vi "CAMERA ROI.vi"(8 "error in (no error)":errorcluster, 11 "Enum":T1=enum."INIT") -> (0 "error out":errorcluster)   [LabVIEW 2025]
uses:
  POST ANALYSIS ENUM.ctl
panel:
  in  "stop":bool
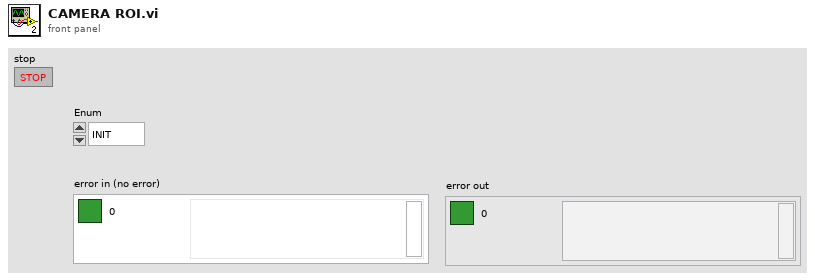
[diagram p1: front panel]
types:
  T1 = typedef "POST ANALYSIS ENUM.ctl" = enum16{"OPEN EXE", "INIT", "OPEN FILE", "FIT", "DRAW REC", "DRAW LINE", "PAN", "ZOOM IN", "ZOOM OUT", "SET ZOOM", "CLEAR ROI", "GET MEASUREMENTS", "RESIZE MODE", "STREAM START", "STREAM STOP", "SHOW UI", "MINIMIZE UI", "HIDE UI", "CKISE APP", "CLOSE CONNECTION", "SAVE IMAGE", "SET ROI COLOR", "READ", "TCP CHECK", "CLOSE"}
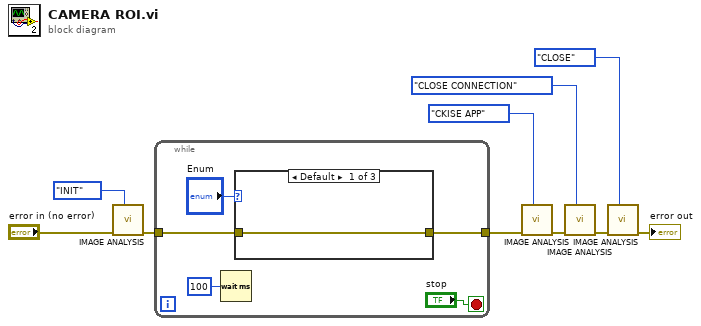
[diagram p0: block diagram]
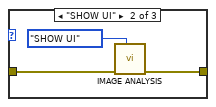
[diagram p2: hidden frame]
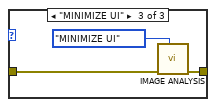
[diagram p3: hidden frame]
diagram:
  n1 = call "IMAGE ANALYSIS.vi"("Enum"=POST_ANALYSIS_ENUM."INIT", "error in"="error in (no error)") -> ("error out"=w9:errorcluster)  [unwired: 8 in, 1 out]
  n2 = while {
    tunnel: w9 -> [w15]
    tunnel: [w14] -> w4
    stop <- "stop" stop-if-true
    n3 = Wait (ms)(milliseconds to wait=u32 100) -> ()  [unwired: 1 out]
    n4 = case shown="Default" "Enum" {
      tunnel: w15 -> [w16 w18 w21]
      tunnel: [w16 w17 w20] -> w14
      frame Default {
      }
      frame "SHOW UI" {
        n5 = call "IMAGE ANALYSIS.vi"("Enum"=POST_ANALYSIS_ENUM."SHOW UI", "error in"=w18) -> ("error out"=w17:errorcluster)  [unwired: 8 in, 1 out]
      }
      frame "MINIMIZE UI" {
        n6 = call "IMAGE ANALYSIS.vi"("Enum"=POST_ANALYSIS_ENUM."MINIMIZE UI", "error in"=w21) -> ("error out"=w20:errorcluster)  [unwired: 8 in, 1 out]
      }
    }
  }
  n7 = call "IMAGE ANALYSIS.vi"("Enum"=POST_ANALYSIS_ENUM."CKISE APP", "error in"=w4) -> ("error out"=w3:errorcluster)  [unwired: 8 in, 1 out]
  n8 = call "IMAGE ANALYSIS.vi"("Enum"=POST_ANALYSIS_ENUM."CLOSE CONNECTION", "error in"=w3) -> ("error out"=w2:errorcluster)  [unwired: 8 in, 1 out]
  n9 = call "IMAGE ANALYSIS.vi"("Enum"=POST_ANALYSIS_ENUM."CLOSE", "error in"=w2) -> ("error out"=→"error out":errorcluster)  [unwired: 8 in, 1 out]
